vi "MTMount_getNextSample_ElevationDrivesThermal.vi"(8 "error in (no error)":errorcluster, 11 "Elevation_Drives_Thermal_Ctl":T1) -> (0 "error out":errorcluster, 2 "function return":i32, 3 "Elevation_Drives_Thermal_Ctl out":T1)   [LabVIEW 2018, in "SALLV_MTMount.lvlib"]
doc: "int MTMount_shm_getNextSample_Elevation_Drives_ThermalLV(MTMount_Elevation_Drives_ThermalLV *Elevation_Drives_Thermal_Ctl );"
uses:
  SALLV_MTMount.lvlib
  DataTypes/Elevation_Drives_Thermal.ctl
  SALLV_MTMount.so
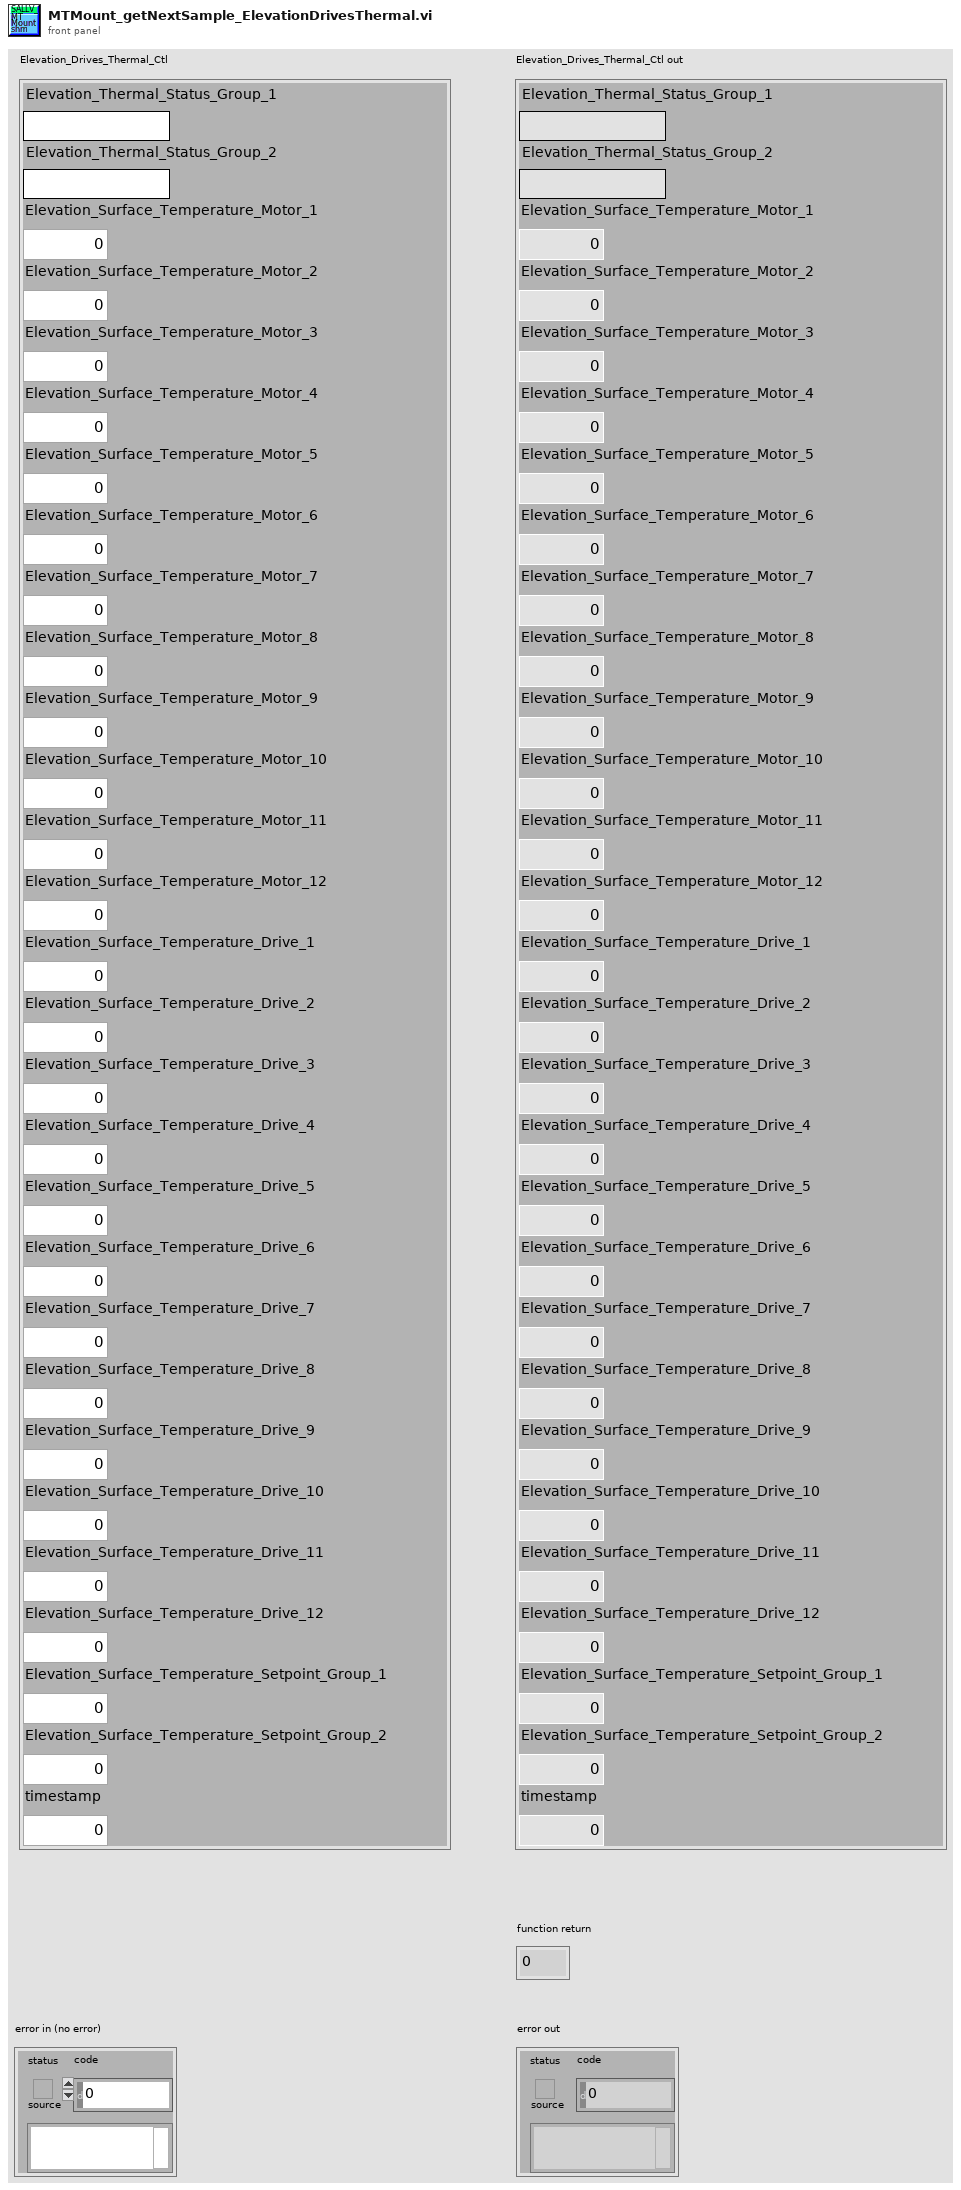
[diagram p1: front panel]
types:
  T1 = typedef "SALLV_MTMount.lvlib/Elevation_Drives_Thermal.ctl" = cluster{"Elevation_Thermal_Status_Group_1":string, "Elevation_Thermal_Status_Group_2":string, "Elevation_Surface_Temperature_Motor_1":dbl, "Elevation_Surface_Temperature_Motor_2":dbl, "Elevation_Surface_Temperature_Motor_3":dbl, "Elevation_Surface_Temperature_Motor_4":dbl, "Elevation_Surface_Temperature_Motor_5":dbl, "Elevation_Surface_Temperature_Motor_6":dbl, "Elevation_Surface_Temperature_Motor_7":dbl, "Elevation_Surface_Temperature_Motor_8":dbl, "Elevation_Surface_Temperature_Motor_9":dbl, "Elevation_Surface_Temperature_Motor_10":dbl, "Elevation_Surface_Temperature_Motor_11":dbl, "Elevation_Surface_Temperature_Motor_12":dbl, "Elevation_Surface_Temperature_Drive_1":dbl, "Elevation_Surface_Temperature_Drive_2":dbl, "Elevation_Surface_Temperature_Drive_3":dbl, "Elevation_Surface_Temperature_Drive_4":dbl, "Elevation_Surface_Temperature_Drive_5":dbl, "Elevation_Surface_Temperature_Drive_6":dbl, "Elevation_Surface_Temperature_Drive_7":dbl, "Elevation_Surface_Temperature_Drive_8":dbl, "Elevation_Surface_Temperature_Drive_9":dbl, "Elevation_Surface_Temperature_Drive_10":dbl, "Elevation_Surface_Temperature_Drive_11":dbl, "Elevation_Surface_Temperature_Drive_12":dbl, "Elevation_Surface_Temperature_Setpoint_Group_1":dbl, "Elevation_Surface_Temperature_Setpoint_Group_2":dbl, "timestamp":dbl}
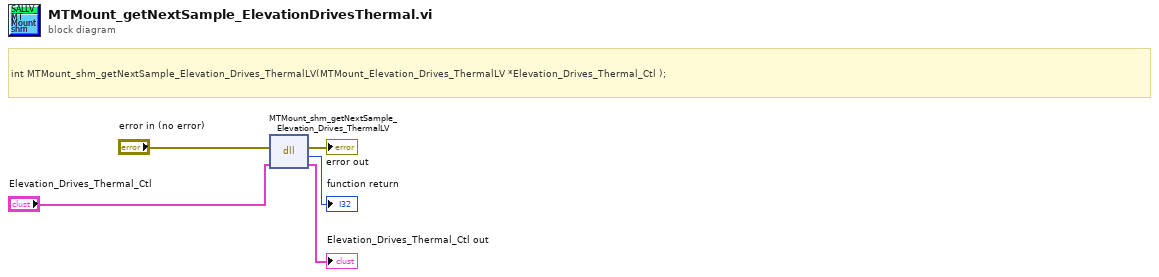
[diagram p0: block diagram]
diagram:
  # "int MTMount_shm_getNextSample_Elevation_Drives_ThermalLV(MTMount_Elevation_Drives_ThermalLV *Elevation_Drives_Thermal_Ctl );"
  n1 = dll-call lib="home/ttsai/Document/salApiMTMount/SALLV_MTMount/SALLV_MTMount.*" fn="MTMount_shm_getNextSample_Elevation_Drives_ThermalLV"(error in="error in (no error)", "Elevation_Drives_Thermal_Ctl"="Elevation_Drives_Thermal_Ctl") -> (error out=→"error out":errorcluster, →"function return":i32, "Elevation_Drives_Thermal_Ctl"=→"Elevation_Drives_Thermal_Ctl out":T1)  [unwired: 2 in, 1 out]
